vi "중점추출.vi"(2 "x,y 배열":cluster{"x":dbl, "y":dbl}[](array[cluster]), 3 "x범위":i32=3000) -> (0 "steer":dbl, 1 "주행 관찰용":cluster{cluster{"x":dbl, "y":dbl}[]}[](array[cluster]))   [LabVIEW 2015]
panel:
  out "XY 그래프":cluster{cluster{"x":dbl, "y":dbl}[]}[](graph)
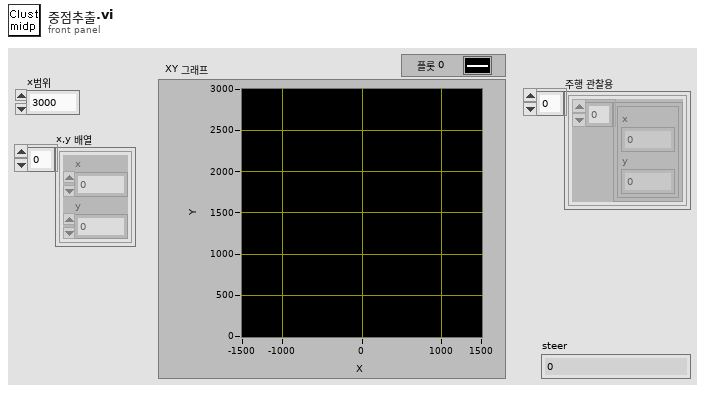
[diagram p1: front panel]
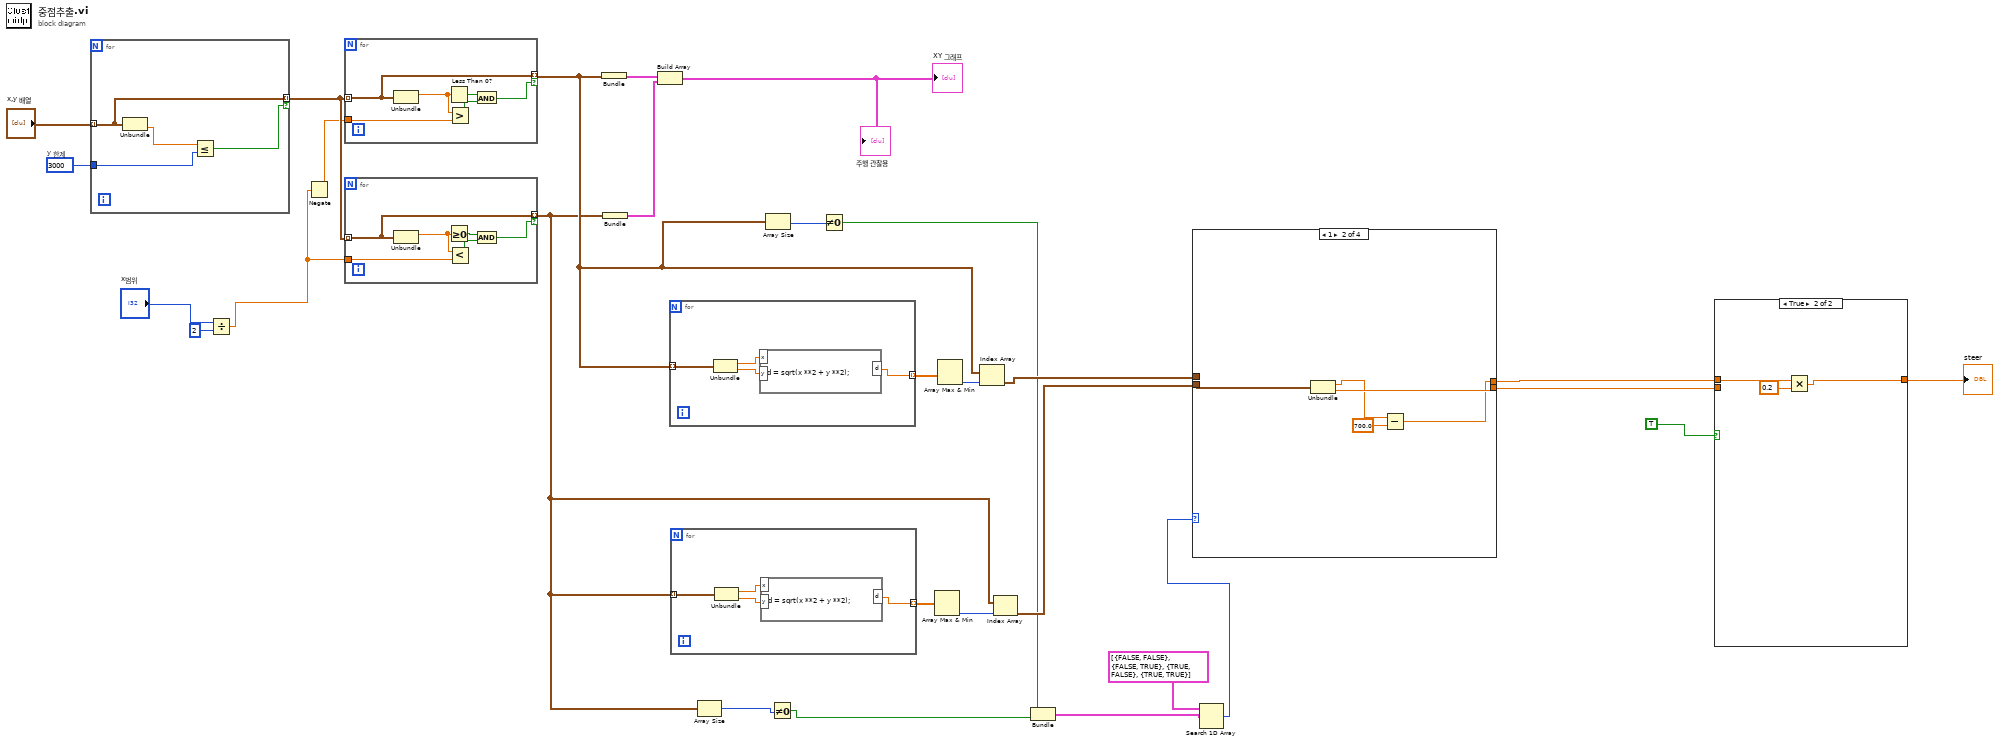
[diagram p0: block diagram]
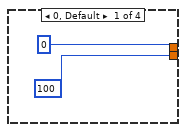
[diagram p2: hidden frame]
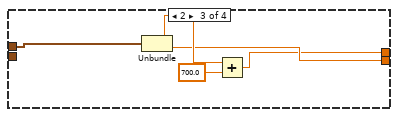
[diagram p3: hidden frame]
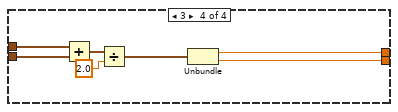
[diagram p4: hidden frame]
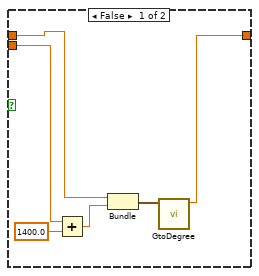
[diagram p5: hidden frame]
diagram:
  w22 = 3000  # y 한계
  n1 = for {
    tunnel: "x,y 배열" -> [w32] mode=indexing
    tunnel: w22 -> [w33]
    tunnel: [w32] -> w21 mode=indexing if=w31
    n2 = Unbundle(w32) -> ("y"=w30:dbl)  [unwired: 1 out]
    n3 = Less Or Equal?(x=w30, y=w33) -> (x <= y?=w31:bool)
  }
  n4 = Divide(x="x범위", y=2) -> (x/y=w11:dbl)
  n5 = Negate(x=w11) -> (-x=w20:dbl)
  n6 = for {
    tunnel: w21 -> [w35] mode=indexing
    tunnel: w20 -> [w36]
    tunnel: [w35] -> w9 mode=indexing if=w34
    n7 = Unbundle(w35) -> ("x"=w37:dbl)  [unwired: 1 out]
    n8 = Less Than 0?(x=w37) -> (x < 0?=w39:bool)
    n9 = Greater?(x=w37, y=w36) -> (0:w38:bool)
    n10 = And(x=w39, y=w38) -> (x .and. y?=w34:bool)
  }
  n11 = for {
    tunnel: w21 -> [w41] mode=indexing
    tunnel: w11 -> [w42]
    tunnel: [w41] -> w8 mode=indexing if=w40
    n12 = Unbundle(w41) -> ("x"=w43:dbl)  [unwired: 1 out]
    n13 = Greater Or Equal To 0?(x=w43) -> (x >= 0?=w45:bool)
    n14 = Less?(x=w43, y=w42) -> (x < y?=w44:bool)
    n15 = And(x=w45, y=w44) -> (x .and. y?=w40:bool)
  }
  n16 = Bundle(w9) -> (w19:cluster{cluster{"x":dbl, "y":dbl}[]})  [unwired: 1 in]
  n17 = Bundle(w8) -> (w18:cluster{cluster{"x":dbl, "y":dbl}[]})  [unwired: 1 in]
  n18 = Build Array(w19, w18) -> (→"XY 그래프" →"주행 관찰용":cluster{cluster{"x":dbl, "y":dbl}[]}[])
  n19 = for {
    tunnel: w9 -> [w47] mode=indexing
    tunnel: [w46] -> w26 mode=indexing
    n20 = Unbundle(w47) -> ("x"=w49:dbl, "y"=w48:dbl)
    n21 = formula code="d = sqrt(x **2 + y **2);"("x"=w49, "y"=w48) -> ("d"=w46:dbl)
  }
  n22 = for {
    tunnel: w8 -> [w51] mode=indexing
    tunnel: [w50] -> w29 mode=indexing
    n23 = Unbundle(w51) -> ("x"=w53:dbl, "y"=w52:dbl)
    n24 = formula code="d = sqrt(x **2 + y **2);"("x"=w53, "y"=w52) -> ("d"=w50:dbl)
  }
  n25 = Array Size(array=w8) -> (size(s)=w7:i32)
  n26 = Array Size(array=w9) -> (size(s)=w6:i32)
  n27 = Not Equal To 0?(x=w7) -> (x != 0?=w4:bool)
  n28 = Not Equal To 0?(x=w6) -> (x != 0?=w5:bool)
  n29 = Array Max & Min(array=w29) -> (min index (indices)=w28:i32)  [unwired: 3 out]
  n30 = Array Max & Min(array=w26) -> (min index (indices)=w25:i32)  [unwired: 3 out]
  n31 = Index Array(array=w9, index=w25) -> (element=w24:cluster{"x":dbl, "y":dbl})
  n32 = Index Array(array=w8, index=w28) -> (element=w27:cluster{"x":dbl, "y":dbl})
  n33 = Bundle(w5, w4) -> (w2:cluster{bool, bool})  [unwired: 1 in]
  n34 = Search 1D Array(1D array=cluster{bool, bool}[] [{FALSE, FALSE}, {FALSE, TRUE}, {TRUE, FALSE}, {TRUE, TRUE}] ("클러스터의 배열 2"), element=w2) -> (index of element=w1:i32)  [unwired: 1 in]
  n35 = case shown="1" w1 {
    tunnel: w27 -> [_ w60 _ w69]
    tunnel: w24 -> [_ _ w63 w68]
    tunnel: [0 w57 w61 w67] -> w16
    tunnel: [100 w59 w62 w66] -> w13
    frame 0, Default {
    }
    frame 1 {
      n36 = Unbundle(w60) -> ("x"=w58:dbl, "y"=w59:dbl)
      n37 = Subtract(x=w58, y=700.0) -> (x-y=w57:dbl)
    }
    frame 2 {
      n38 = Unbundle(w63) -> ("x"=w65:dbl, "y"=w62:dbl)
      n39 = Add(x=w65, y=700.0) -> (x+y=w61:dbl)
    }
    frame 3 {
      n40 = Add(x=w68, y=w69) -> (x+y=w71:cluster{"x":dbl, "y":dbl})
      n41 = Divide(x=w71, y=2.0) -> (x/y=w70:cluster{"x":dbl, "y":dbl})
      n42 = Unbundle(w70) -> ("x"=w67:dbl, "y"=w66:dbl)
    }
  }
  n43 = case shown="True" TRUE {
    tunnel: w16 -> [w78 w81]
    tunnel: [w73 w79] -> w15
    tunnel: w13 -> [w76 _]
    frame False {
      n44 = Add(x=w76, y=1400.0) -> (x+y=w77:dbl)
      n45 = Bundle("x"=w78, w77) -> (w74:cluster{"x":dbl, dbl})  [unwired: 1 in]
      n46 = call "GtoDegree.vi"("PathPointG"=w74) -> ("steer"=w73:dbl)  [unwired: 10 in]
    }
    frame True {
      n47 = Multiply(x=w81, y=0.2) -> (x*y=w79:dbl)
    }
  }
  "steer" <- w15
